vi "Resolve Drive Letter To Mapped Path.vi"(0 "Drive Letter":string, 11 "error in (no error)":errorcluster) -> (4 "Mapped Path":path, 6 "Found":bool, 15 "error out":errorcluster)   [LabVIEW 2017, in "G3_Build Process File Utilities.lvlib"]
uses:
  G3_Build Process File Utilities.lvlib
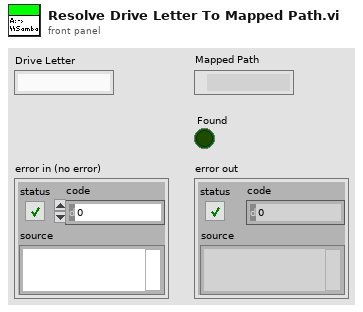
[diagram p1: front panel]
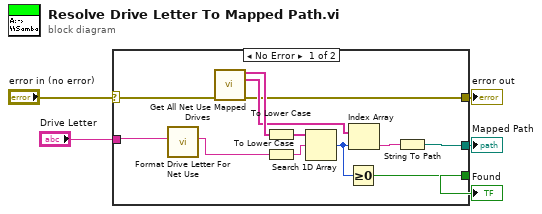
[diagram p0: block diagram]
diagram:
  n1 = case shown="No Error" "error in (no error)" {
    selector: "error in (no error)" -> [w14 w18]
    tunnel: "Drive Letter" -> [w7 _]
    tunnel: [w8 _] -> w4
    tunnel: [w13 w18] -> w2
    tunnel: [w11 _] -> w1
    frame No Error {
      n2 = call "Format Drive Letter For Net Use.vi"("Drive Letter"=w7) -> ("String"=w6:string)  [unwired: 10 in]
      n3 = call "Get All Net Use Mapped Drives.vi"("error in (no error)"=w14) -> ("Mapped Drive Letters"=w17:string[], "Mapped Paths"=w16:string[], "error out"=w13:errorcluster)  [unwired: 12 in]
      n4 = To Lower Case(string=w17) -> (all lower case string=w10:string[])
      n5 = To Lower Case(string=w6) -> (all lower case string=w9:string)
      n6 = Search 1D Array(1D array=w10, element=w9) -> (index of element=w12:i32)  [unwired: 1 in]
      n7 = Greater Or Equal To 0?(x=w12) -> (x >= 0?=w11:bool)
      n8 = Index Array(array=w16, index=w12) -> (element=w15:string)
      n9 = String To Path(string=w15) -> (path=w8:path)
    }
    frame Error {
    }
  }
  "Mapped Path" <- w4
  "error out" <- w2
  "Found" <- w1
